vi "rx_ceEq.vi"(2 "preamble":cdb[](array[numeric])=[-0.7071067811865475+0.7071067811865476i, 0.7071067811865476+0.7071067811865475i, 0.7071067811865474-0.7071067811865477i, 0.7071067811865476+0.7071067811865475i, -0.7071067811865475+0.7071067811865476i, -0.7071067811865477-0.7071067811865475i, 0.7071067811865476+0.7071067811865475i, -0.7071067811865477-0.7071067811865475i, -0.7071067811865475+0.7071067811865476i, 0.7071067811865476+0.7071067811865475i, 0.7071067811865474-0.7071067811865477i, 0.7071067811865476+0.7071067811865475i, -0.7071067811865475+0.7071067811865476i, -0.7071067811865477-0.7071067811865475i, 0.7071067811865476+0.7071067811865475i, -0.7071067811865477-0.7071067811865475i, -0.7071067811865475+0.7071067811865476i, 0.7071067811865476+0.7071067811865475i, 0.7071067811865474-0.7071067811865477i, 0.7071067811865476+0.7071067811865475i, -0.7071067811865475+0.7071067811865476i, -0.7071067811865477-0.7071067811865475i, 0.7071067811865476+0.7071067811865475i, -0.7071067811865477-0.7071067811865475i, -0.7071067811865475+0.7071067811865476i, 0.7071067811865476+0.7071067811865475i, 0.7071067811865474-0.7071067811865477i, 0.7071067811865476+0.7071067811865475i, -0.7071067811865475+0.7071067811865476i, -0.7071067811865477-0.7071067811865475i, 0.7071067811865476+0.7071067811865475i, -0.7071067811865477-0.7071067811865475i, -0.7071067811865475+0.7071067811865476i, 0.7071067811865476+0.7071067811865475i, 0.7071067811865474-0.7071067811865477i, 0.7071067811865476+0.7071067811865475i, -0.7071067811865475+0.7071067811865476i, -0.7071067811865477-0.7071067811865475i, 0.7071067811865476+0.7071067811865475i, -0.7071067811865477-0.7071067811865475i, -0.7071067811865475+0.7071067811865476i, 0.7071067811865476+0.7071067811865475i, 0.7071067811865474-0.7071067811865477i, 0.7071067811865476+0.7071067811865475i, -0.7071067811865475+0.7071067811865476i, -0.7071067811865477-0.7071067811865475i, 0.7071067811865476+0.7071067811865475i, -0.7071067811865477-0.7071067811865475i, -0.7071067811865475+0.7071067811865476i, 0.7071067811865476+0.7071067811865475i, 0.7071067811865474-0.7071067811865477i, 0.7071067811865476+0.7071067811865475i, -0.7071067811865475+0.7071067811865476i, -0.7071067811865477-0.7071067811865475i, 0.7071067811865476+0.7071067811865475i, -0.7071067811865477-0.7071067811865475i, -0.7071067811865475+0.7071067811865476i, 0.7071067811865476+0.7071067811865475i, 0.7071067811865474-0.7071067811865477i, 0.7071067811865476+0.7071067811865475i, -0.7071067811865475+0.7071067811865476i, -0.7071067811865477-0.7071067811865475i, 0.7071067811865476+0.7071067811865475i, -0.7071067811865477-0.7071067811865475i], 3 "symbols":cdb[](array[numeric])) -> (0 "valid?":bool, 1 "eq symbols":cdb[](array[numeric]))   [LabVIEW 2014]
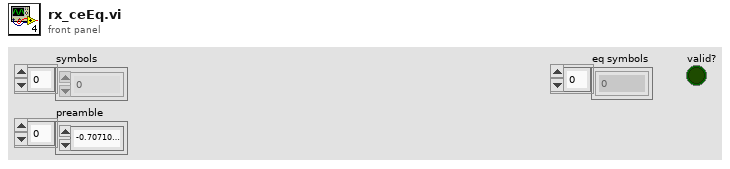
[diagram p1: front panel]
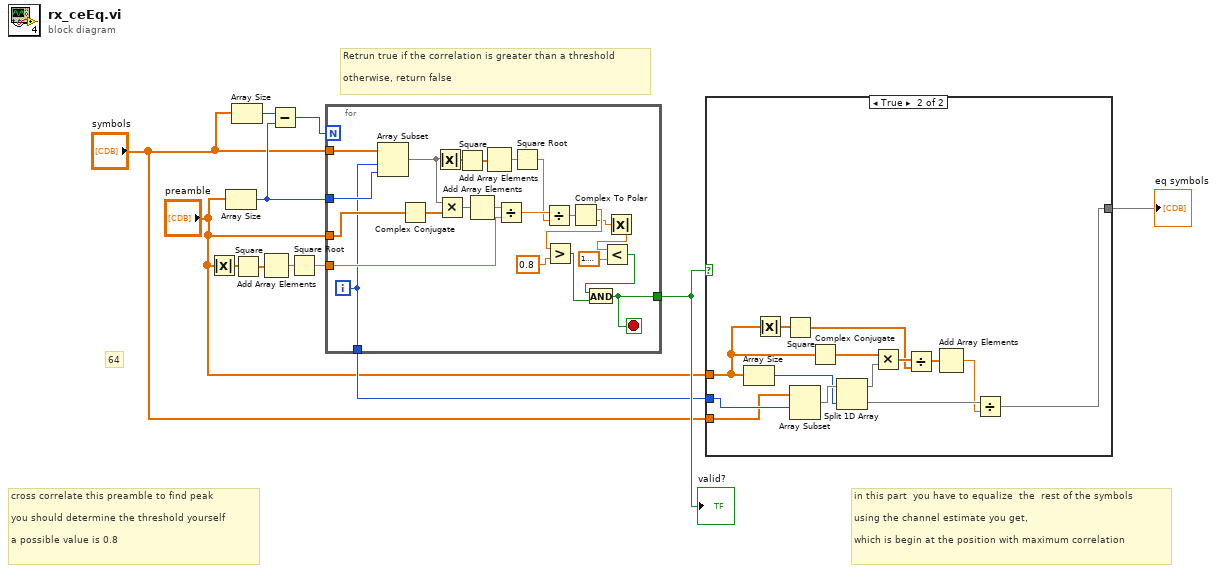
[diagram p0: block diagram]
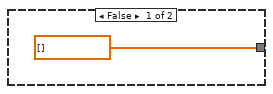
[diagram p2: hidden frame]
diagram:
  # "in this part  you have to equalize  the  rest of the symbols\n\nusing the channel estimate you get, \n\nwhich is begin at the position with maximum correlation"
  # "Retrun true if the correlation is greater than a threshold\n\notherwise, return false"
  # "cross correlate this preamble to find peak \n\nyou should determine the threshold yourself\n\na possible value is 0.8"
  # "64"
  n1 = Absolute Value(x="preamble") -> (abs(x)=w8:dbl[])
  n2 = Array Size(array="preamble") -> (size(s)=w5:i32)
  n3 = Array Size(array="symbols") -> (size(s)=w6:i32)
  n4 = Square(x=w8) -> (x^2=w11:dbl[])
  n5 = Add Array Elements(numeric array=w11) -> (sum=w10:dbl)
  n6 = Subtract(x=w6, y=w5) -> (x-y=w4:i32)
  n7 = Square Root(x=w10) -> (sqrt(x)=w9:dbl)
  n8 = for {
    N: w4 -> [_]
    tunnel: "symbols" -> [w35]
    tunnel: w5 -> [w34]
    tunnel: "preamble" -> [w28]
    tunnel: w9 -> [w26]
    tunnel: [w14] -> w7
    tunnel: [w13] -> w3
    i -> [w13]
    stop <- w14 stop-if-true
    n9 = Array Subset(array=w35, index=w13, length=w34) -> (w30:cdb[])
    n10 = Complex Conjugate(1:w28) -> (0:w29:cdb[])
    n11 = Absolute Value(x=w30) -> (abs(x)=w22:dbl[])
    n12 = Multiply(x=w30, y=w29) -> (x*y=w33:cdb[])
    n13 = Square(x=w22) -> (x^2=w32:dbl[])
    n14 = Add Array Elements(numeric array=w33) -> (sum=w27:cdb)
    n15 = Add Array Elements(numeric array=w32) -> (sum=w31:dbl)
    n16 = Divide(x=w27, y=w26) -> (x/y=w25:cdb)
    n17 = Square Root(x=w31) -> (sqrt(x)=w24:dbl)
    n18 = Divide(x=w25, y=w24) -> (x/y=w21:cdb)
    n19 = Complex To Polar(r * e^(i*theta)=w21) -> (r=w20:dbl, theta=w19:dbl)
    n20 = Greater?(x=w20, y=0.8) -> (0:w15:bool)
    n21 = Absolute Value(x=w19) -> (abs(x)=w18:dbl)
    n22 = Less?(x=w18, y=1.5707963267948966) -> (x < y?=w16:bool)
    n23 = And(x=w16, y=w15) -> (x .and. y?=w14:bool)
  }
  "valid?" <- w7
  n24 = case shown="True" w7 {
    tunnel: [cdb[] [] w37] -> w12
    tunnel: w3 -> [_ w50]
    tunnel: "preamble" -> [_ w46]
    tunnel: "symbols" -> [_ w49]
    frame False {
    }
    frame True {
      n25 = Array Size(array=w46) -> (size(s)=w41:i32)
      n26 = Absolute Value(x=w46) -> (abs(x)=w47:dbl[])
      n27 = Square(x=w47) -> (x^2=w44:dbl[])
      n28 = Array Subset(array=w49, index=w50) -> (w42:cdb[])  [unwired: 1 in]
      n29 = Complex Conjugate(1:w46) -> (0:w48:cdb[])
      n30 = Split 1D Array(array=w42, index=w41) -> (first subarray=w40:cdb[], second subarray=w39:cdb[])
      n31 = Multiply(x=w48, y=w40) -> (x*y=w45:cdb[])
      n32 = Divide(x=w45, y=w44) -> (x/y=w43:cdb[])
      n33 = Add Array Elements(numeric array=w43) -> (sum=w38:cdb)
      n34 = Divide(x=w39, y=w38) -> (x/y=w37:cdb[])
    }
  }
  "eq symbols" <- w12
